vi "remove hidden points.vi"(8 "error in (no error)":errorcluster, 9 "Y Array in":dbl[](array[numeric]), 10 "X Array In":dbl[](array[numeric]), 11 "XYGraph in":refnum<vi>) -> (0 "error out":errorcluster, 1 "Y Array out":dbl[](array[numeric]), 2 "X Array Out":dbl[](array[numeric]))   [LabVIEW 2013, in "Manipulate IPF.lvlib"]
uses:
  Manipulate IPF.lvlib
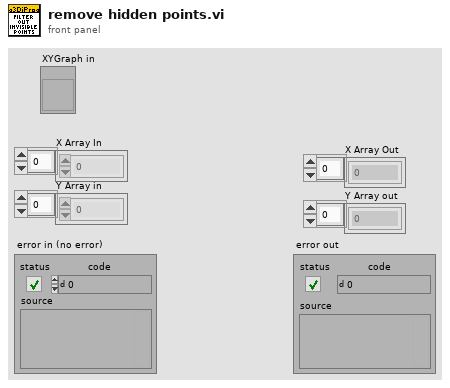
[diagram p1: front panel]
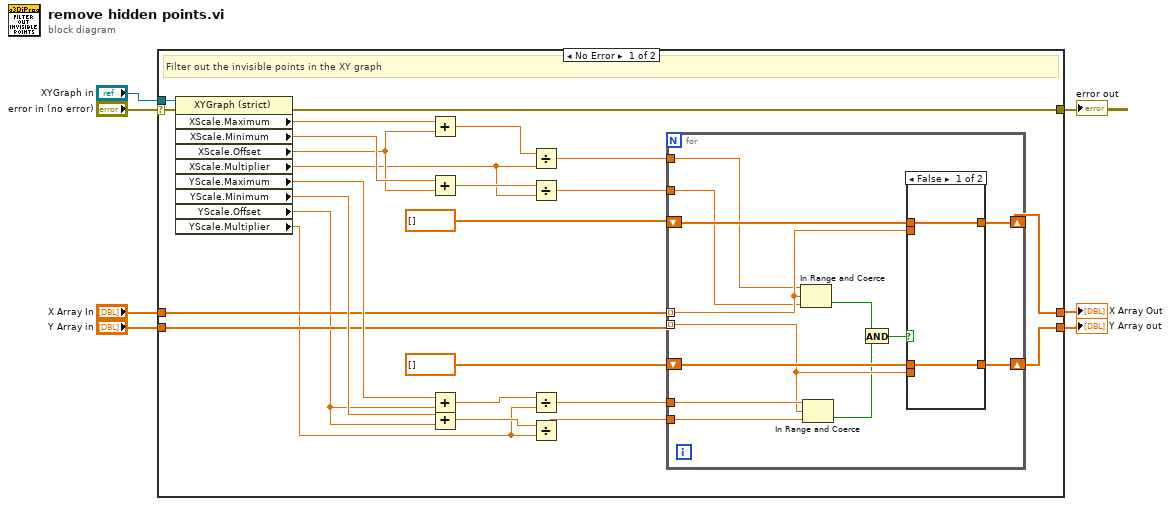
[diagram p0: block diagram]
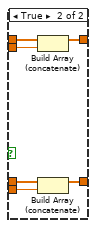
[diagram p2: hidden frame]
diagram:
  n1 = case shown="No Error" "error in (no error)" {
    selector: "error in (no error)" -> [w27 w56]
    tunnel: "XYGraph in" -> [w28 _]
    tunnel: [w26 w56] -> w5
    tunnel: "X Array In" -> [w23 w55]
    tunnel: "Y Array in" -> [w22 w54]
    tunnel: [w21 w55] -> w2
    tunnel: [w20 w54] -> w1
    frame No Error {
      # "Filter out the invisible points in the XY graph"
      n2 = property class="XYGraph (strict)"(reference=w28, error in=w27) -> (error out=w26:errorcluster, "XScale.Maximum"=w30:dbl, "XScale.Minimum"=w29:dbl, "XScale.Offset"=w19:dbl, "XScale.Multiplier"=w15:dbl, "YScale.Maximum"=w25:dbl, "YScale.Minimum"=w24:dbl, "YScale.Offset"=w18:dbl, "YScale.Multiplier"=w9:dbl)  [unwired: 1 out]
      n3 = Add(x=w30, y=w19) -> (x+y=w17:dbl)
      n4 = Add(x=w29, y=w19) -> (x+y=w16:dbl)
      n5 = Add(x=w25, y=w18) -> (x+y=w12:dbl)
      n6 = Add(x=w24, y=w18) -> (x+y=w10:dbl)
      n7 = Divide(x=w17, y=w15) -> (x/y=w14:dbl)
      n8 = Divide(x=w16, y=w15) -> (x/y=w13:dbl)
      n9 = Divide(x=w12, y=w9) -> (x/y=w11:dbl)
      n10 = Divide(x=w10, y=w9) -> (x/y=w8:dbl)
      n11 = for {
        tunnel: w22 -> [w36] mode=indexing
        tunnel: w23 -> [w41] mode=indexing
        shift-right: [w45] -> w21
        shift-left: dbl[] [] -> [w44]
        shift-right: [w42] -> w20
        shift-left: dbl[] [] -> [w43]
        tunnel: w14 -> [w40]
        tunnel: w13 -> [w39]
        tunnel: w11 -> [w38]
        tunnel: w8 -> [w37]
        n12 = In Range and Coerce(upper limit=w40, x=w41, lower limit=w39) -> (In Range?=w35:bool)  [unwired: 1 out]
        n13 = In Range and Coerce(upper limit=w38, x=w36, lower limit=w37) -> (In Range?=w34:bool)  [unwired: 1 out]
        n14 = And(x=w35, y=w34) -> (x .and. y?=w33:bool)
        n15 = case shown="False" w33 {
          tunnel: [w47 w53] -> w45
          tunnel: w44 -> [w47 w52]
          tunnel: w41 -> [_ w51]
          tunnel: w43 -> [w46 w50]
          tunnel: [w46 w49] -> w42
          tunnel: w36 -> [_ w48]
          frame False {
          }
          frame True {
            n16 = Build Array (concatenate)(w52, w51) -> (w53:dbl[])
            n17 = Build Array (concatenate)(w50, w48) -> (w49:dbl[])
          }
        }
      }
    }
    frame Error {
    }
  }
  "error out" <- w5
  "X Array Out" <- w2
  "Y Array out" <- w1
